vi "Set-Get-Avg_PM.vi"(0 "instrument handle":refnum<visa-resource-name>, 5 "Average Time (0.0)":dbl, 7 "Sensor":string, 9 "Average Count":i32=1 min=1 step=1, 11 "error in (no error)":errorcluster {"code" format="%.0x"}) -> (4 "instrument handle out":refnum<visa-resource-name>, 6 "Average Time":dbl, 8 "Sensor 2":string, 10 "Average Count":i32=1 min=1 step=1, 15 "error out":errorcluster)   [LabVIEW 2018]
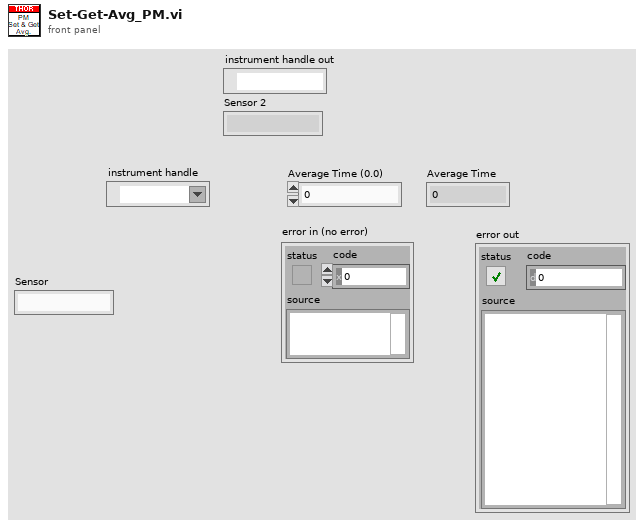
[diagram p1: front panel]
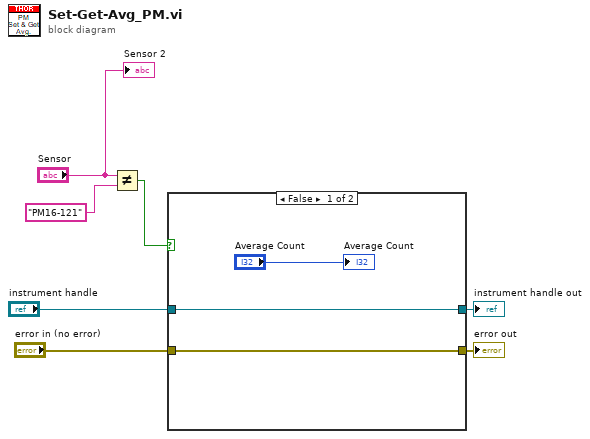
[diagram p0: block diagram]
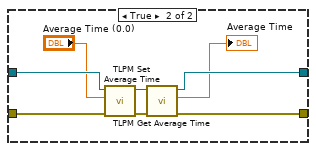
[diagram p2: hidden frame]
diagram:
  n1 = Not Equal?(x="Sensor", y="PM16-121") -> (x != y?=w1:bool)
  n2 = case shown="False" w1 {
    tunnel: "instrument handle" -> [w10 w18]
    tunnel: "error in (no error)" -> [w9 w17]
    tunnel: [w9 w16] -> w5
    tunnel: [w10 w15] -> w4
    frame False {
      "Average Count" <- "Average Count"
    }
    frame True {
      n3 = call "TLPM Set Average Time.vi"("error in (no error)"=w17, "Average Time (0.0)"="Average Time (0.0)", "instrument handle"=w18) -> ("error out"=w13:errorcluster, "instrument handle out"=w14:refnum<visa-resource-name>)  [unwired: 7 in]
      n4 = call "TLPM Get Average Time.vi"("error in (no error)"=w13, "instrument handle"=w14) -> ("error out"=w16:errorcluster, "Average Time"=→"Average Time":dbl, "instrument handle out"=w15:refnum<visa-resource-name>)  [unwired: 7 in]
    }
  }
  "error out" <- w5
  "instrument handle out" <- w4
  "Sensor 2" <- "Sensor"
